vi "new FGGA TCP Packet_v3.1.vi"(0 "ID":string, 5 "Version":string, 7 "TCP Packet In":string, 9 "utc_time":u32, 12 "Data Array":string[](array[string])) -> (8 "TCP Binary Packet":string)   [LabVIEW 2014]
panel:
  out "array":string[](array[string])
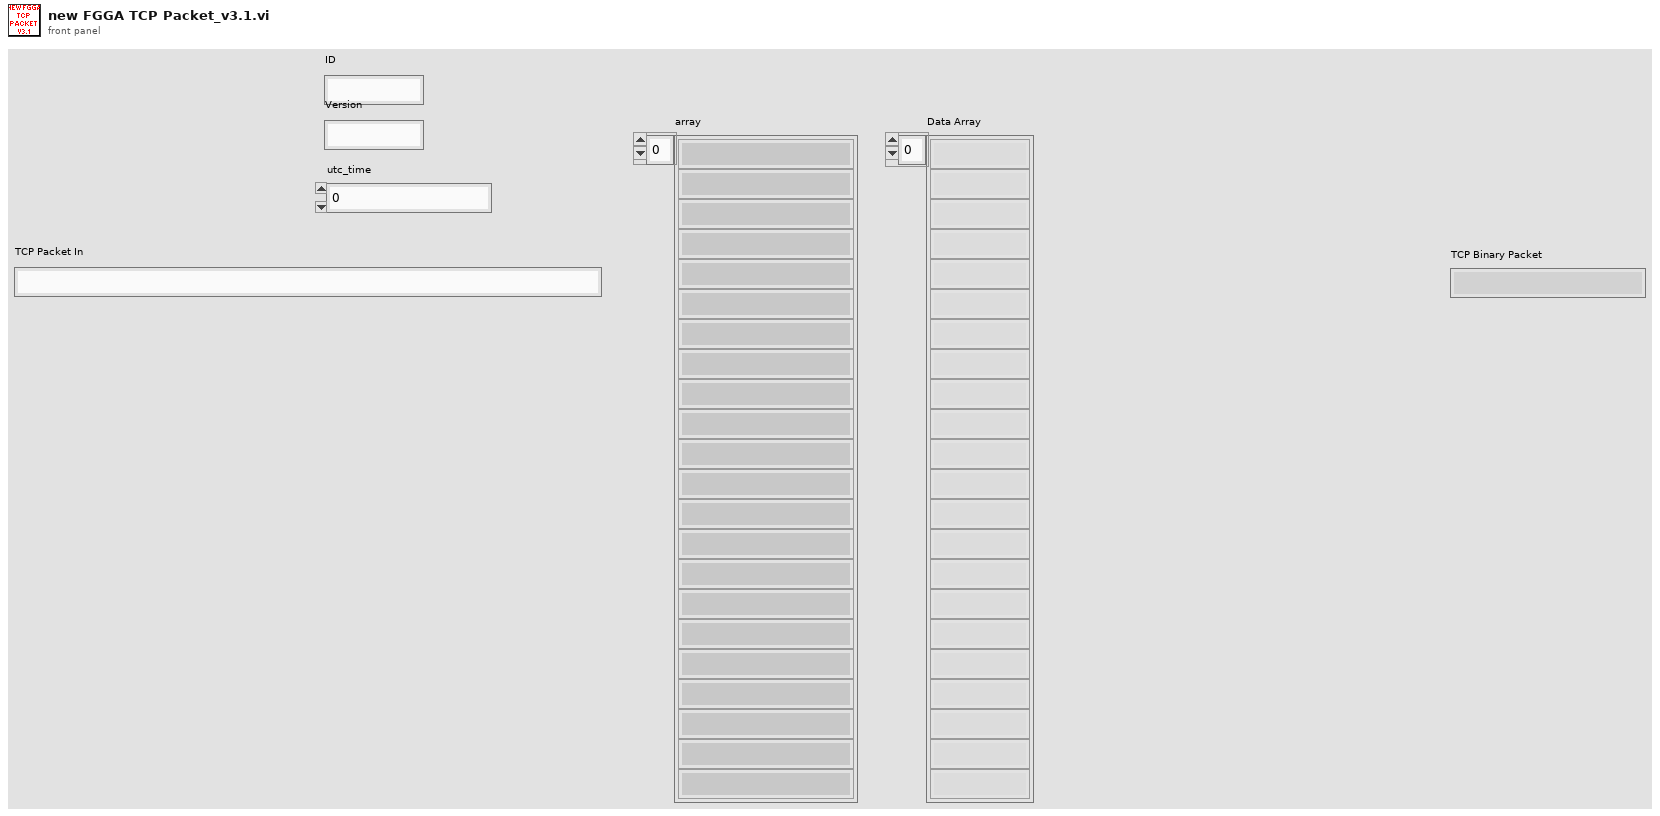
[diagram p1: front panel]
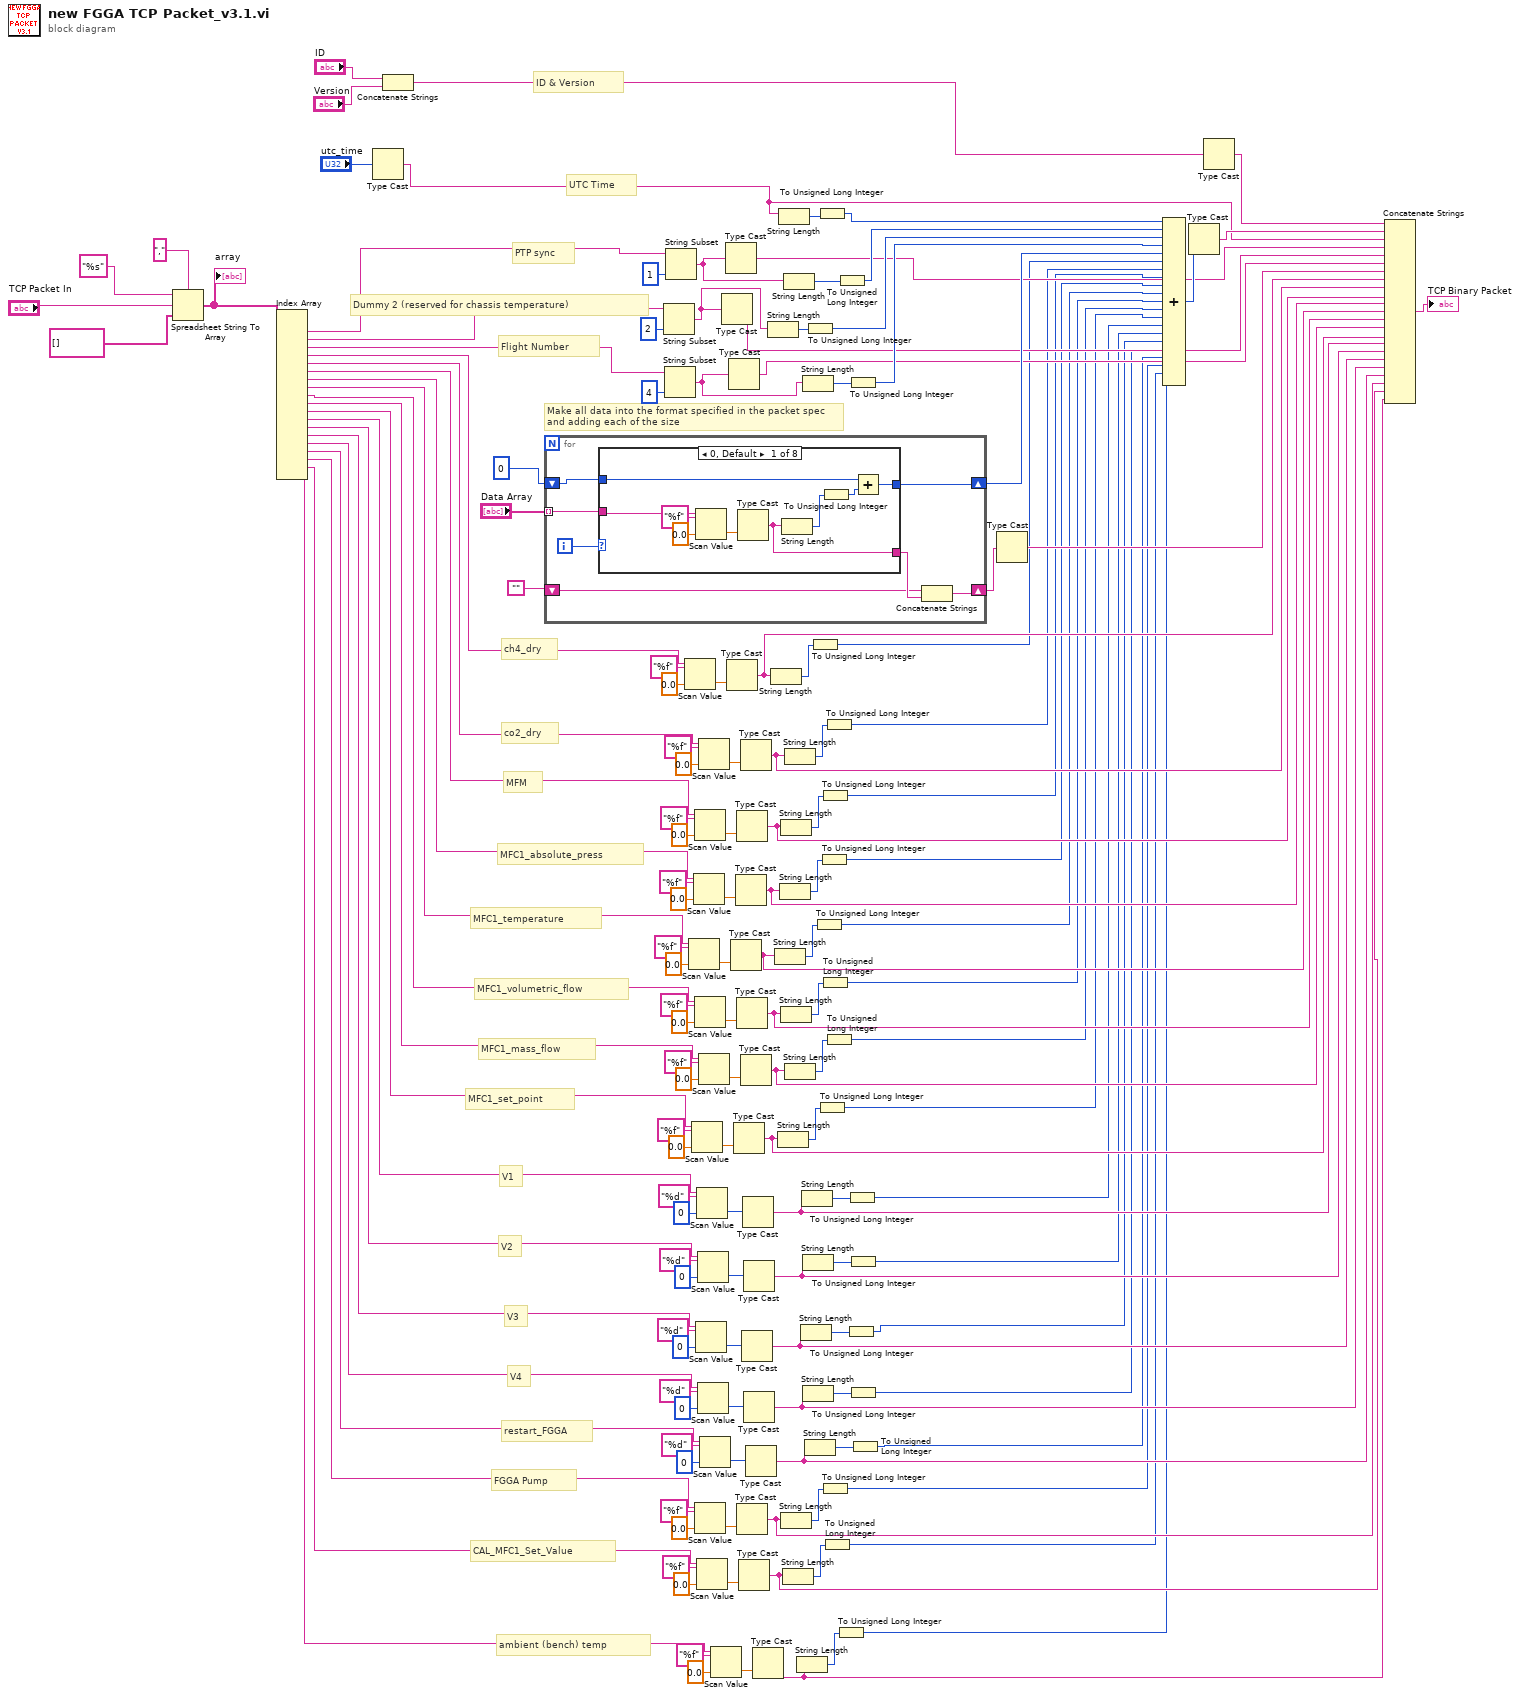
[diagram p0: block diagram]
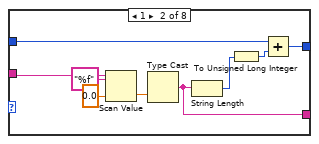
[diagram p2: hidden frame]
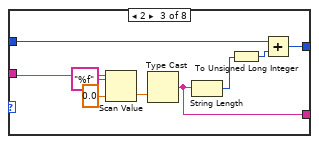
[diagram p3: hidden frame]
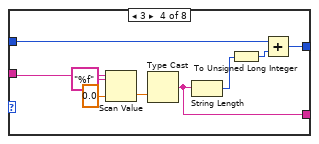
[diagram p4: hidden frame]
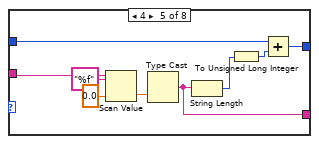
[diagram p5: hidden frame]
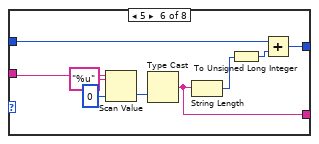
[diagram p6: hidden frame]
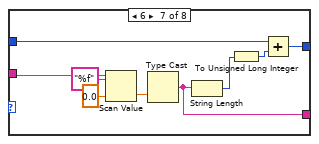
[diagram p7: hidden frame]
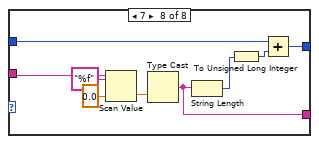
[diagram p8: hidden frame]
diagram:
  # "ambient (bench) temp"
  # "PTP sync"
  # "CAL_MFC1_Set_Value"
  # "FGGA Pump"
  # "restart_FGGA"
  # "V4"
  # "V3"
  # "V2"
  # "V1"
  # "MFC1_set_point"
  # "MFC1_mass_flow"
  # "MFC1_volumetric_flow"
  # "MFC1_temperature"
  # "MFC1_absolute_press"
  # "MFM"
  # "co2_dry"
  # "ch4_dry"
  # "Flight Number"
  # "Dummy 2 (reserved for chassis temperature)"
  # "UTC Time"
  # "ID & Version"
  # "Make all data into the format specified in the packet spec\nand adding each of the size"
  n1 = Spreadsheet String To Array(delimiter (Tab)=",", format string="%s", spreadsheet string="TCP Packet In", array type (2D Dbl)=string[] []) -> (array=w109:string[])
  "array" <- w109
  n2 = Index Array(array=w109) -> (element #1=w108:string, element #2=w107:string, element #3=w106:string, element #4=w105:string, element #5=w104:string, element #6=w79:string, element #7=w76:string, element #8=w73:string, element #9=w70:string, element #10=w67:string, element #11=w64:string, element #12=w57:string, element #13=w50:string, element #14=w27:string, element #15=w24:string, element #16=w21:string, element #17=w18:string, element #18=w15:string, element #19=w3:string)  [unwired: 19 in]
  n3 = Type Cast(x="utc_time") -> (*(type *) &x=w8:string)  [unwired: 1 in]
  n4 = Concatenate Strings("ID", "Version") -> (w10:string)
  n5 = for {
    tunnel: "Data Array" -> [w158] mode=indexing
    shift-right: [w156] -> w140
    shift-left: u32 0 -> [w157]
    shift-right: [w155] -> w129
    shift-left: "" -> [w153]
    i -> [w159]
    n6 = case shown="0, Default" w159 {
      tunnel: w158 -> [w166 w175 w184 w193 w202 w211 w220 w229]
      tunnel: w157 -> [w164 w173 w182 w191 w200 w209 w218 w227]
      tunnel: [w161 w170 w179 w188 w197 w206 w215 w224] -> w156
      tunnel: [w160 w169 w178 w187 w196 w205 w214 w223] -> w154
      frame 0, Default {
        n7 = Scan Value(string=w166, format string="%f", default (0 dbl)=sgl 0.0 ("default (0 I32)")) -> (value=w168:sgl)  [unwired: 1 out]
        n8 = Type Cast(x=w168) -> (*(type *) &x=w160:string)  [unwired: 1 in]
        n9 = String Length(string=w160) -> (length=w163:i32)
        n10 = To Unsigned Long Integer(number=w163) -> (unsigned 32bit integer=w162:u32)
        n11 = Add(x=w164, y=w162) -> (x+y=w161:u32)
      }
      frame 1 {
        n12 = Scan Value(string=w175, format string="%f", default (0 dbl)=sgl 0.0 ("default (0 I32)")) -> (value=w177:sgl)  [unwired: 1 out]
        n13 = Type Cast(x=w177) -> (*(type *) &x=w169:string)  [unwired: 1 in]
        n14 = String Length(string=w169) -> (length=w172:i32)
        n15 = To Unsigned Long Integer(number=w172) -> (unsigned 32bit integer=w171:u32)
        n16 = Add(x=w173, y=w171) -> (x+y=w170:u32)
      }
      frame 2 {
        n17 = Scan Value(string=w184, format string="%f", default (0 dbl)=sgl 0.0 ("default (0 I32)")) -> (value=w186:sgl)  [unwired: 1 out]
        n18 = Type Cast(x=w186) -> (*(type *) &x=w178:string)  [unwired: 1 in]
        n19 = String Length(string=w178) -> (length=w181:i32)
        n20 = To Unsigned Long Integer(number=w181) -> (unsigned 32bit integer=w180:u32)
        n21 = Add(x=w182, y=w180) -> (x+y=w179:u32)
      }
      frame 3 {
        n22 = Scan Value(string=w193, format string="%f", default (0 dbl)=sgl 0.0 ("default (0 I32)")) -> (value=w195:sgl)  [unwired: 1 out]
        n23 = Type Cast(x=w195) -> (*(type *) &x=w187:string)  [unwired: 1 in]
        n24 = String Length(string=w187) -> (length=w190:i32)
        n25 = To Unsigned Long Integer(number=w190) -> (unsigned 32bit integer=w189:u32)
        n26 = Add(x=w191, y=w189) -> (x+y=w188:u32)
      }
      frame 4 {
        n27 = Scan Value(string=w202, format string="%f", default (0 dbl)=sgl 0.0 ("default (0 I32)")) -> (value=w204:sgl)  [unwired: 1 out]
        n28 = Type Cast(x=w204) -> (*(type *) &x=w196:string)  [unwired: 1 in]
        n29 = String Length(string=w196) -> (length=w199:i32)
        n30 = To Unsigned Long Integer(number=w199) -> (unsigned 32bit integer=w198:u32)
        n31 = Add(x=w200, y=w198) -> (x+y=w197:u32)
      }
      frame 5 {
        n32 = Scan Value(string=w211, format string="%u", default (0 dbl)=u16 0 ("default (0 I32)")) -> (value=w213:u16)  [unwired: 1 out]
        n33 = Type Cast(x=w213) -> (*(type *) &x=w205:string)  [unwired: 1 in]
        n34 = String Length(string=w205) -> (length=w208:i32)
        n35 = To Unsigned Long Integer(number=w208) -> (unsigned 32bit integer=w207:u32)
        n36 = Add(x=w209, y=w207) -> (x+y=w206:u32)
      }
      frame 6 {
        n37 = Scan Value(string=w220, format string="%f", default (0 dbl)=sgl 0.0 ("default (0 I32)")) -> (value=w222:sgl)  [unwired: 1 out]
        n38 = Type Cast(x=w222) -> (*(type *) &x=w214:string)  [unwired: 1 in]
        n39 = String Length(string=w214) -> (length=w217:i32)
        n40 = To Unsigned Long Integer(number=w217) -> (unsigned 32bit integer=w216:u32)
        n41 = Add(x=w218, y=w216) -> (x+y=w215:u32)
      }
      frame 7 {
        n42 = Scan Value(string=w229, format string="%f", default (0 dbl)=sgl 0.0 ("default (0 I32)")) -> (value=w231:sgl)  [unwired: 1 out]
        n43 = Type Cast(x=w231) -> (*(type *) &x=w223:string)  [unwired: 1 in]
        n44 = String Length(string=w223) -> (length=w226:i32)
        n45 = To Unsigned Long Integer(number=w226) -> (unsigned 32bit integer=w225:u32)
        n46 = Add(x=w227, y=w225) -> (x+y=w224:u32)
      }
    }
    n47 = Concatenate Strings(w153, w154) -> (w155:string)
  }
  n48 = String Subset(string=w107, length (rest)=2 ("length (rest)")) -> (substring=w127:string)  [unwired: 1 in]
  n49 = String Subset(string=w106, length (rest)=4 ("length (rest)")) -> (substring=w133:string)  [unwired: 1 in]
  n50 = String Subset(string=w108, length (rest)=1 ("length (rest)")) -> (substring=w136:string)  [unwired: 1 in]
  n51 = Scan Value(string=w105, format string="%f", default (0 dbl)=sgl 0.0 ("default (0 I32)")) -> (value=w125:sgl)  [unwired: 1 out]
  n52 = Scan Value(string=w73, format string="%f", default (0 dbl)=sgl 0.0 ("default (0 I32)")) -> (value=w95:sgl)  [unwired: 1 out]
  n53 = Scan Value(string=w64, format string="%f", default (0 dbl)=sgl 0.0 ("default (0 I32)")) -> (value=w83:sgl)  [unwired: 1 out]
  n54 = Scan Value(string=w76, format string="%f", default (0 dbl)=sgl 0.0 ("default (0 I32)")) -> (value=w99:sgl)  [unwired: 1 out]
  n55 = Scan Value(string=w79, format string="%f", default (0 dbl)=sgl 0.0 ("default (0 I32)")) -> (value=w103:sgl)  [unwired: 1 out]
  n56 = Scan Value(string=w70, format string="%f", default (0 dbl)=sgl 0.0 ("default (0 I32)")) -> (value=w91:sgl)  [unwired: 1 out]
  n57 = Scan Value(string=w18, format string="%f", default (0 dbl)=sgl 0.0 ("default (0 I32)")) -> (value=w35:sgl)  [unwired: 1 out]
  n58 = Scan Value(string=w27, format string="%d", default (0 dbl)=u16 0 ("default (0 I32)")) -> (value=w44:u16)  [unwired: 1 out]
  n59 = Scan Value(string=w57, format string="%d", default (0 dbl)=u16 0 ("default (0 I32)")) -> (value=w58:u16)  [unwired: 1 out]
  n60 = Scan Value(string=w15, format string="%f", default (0 dbl)=sgl 0.0 ("default (0 I32)")) -> (value=w31:sgl)  [unwired: 1 out]
  n61 = Scan Value(string=w50, format string="%d", default (0 dbl)=u16 0 ("default (0 I32)")) -> (value=w51:u16)  [unwired: 1 out]
  n62 = Scan Value(string=w24, format string="%d", default (0 dbl)=u16 0 ("default (0 I32)")) -> (value=w40:u16)  [unwired: 1 out]
  n63 = Scan Value(string=w104, format string="%f", default (0 dbl)=sgl 0.0 ("default (0 I32)")) -> (value=w119:sgl)  [unwired: 1 out]
  n64 = Scan Value(string=w67, format string="%f", default (0 dbl)=sgl 0.0 ("default (0 I32)")) -> (value=w87:sgl)  [unwired: 1 out]
  n65 = Scan Value(string=w21, format string="%d", default (0 dbl)=u16 0 ("default (0 I32)")) -> (value=w36:u16)  [unwired: 1 out]
  n66 = Scan Value(string=w3, format string="%f", default (0 dbl)=sgl 0.0 ("default (0 I32)")) -> (value=w7:sgl)  [unwired: 1 out]
  n67 = Type Cast(x=w127) -> (*(type *) &x=w126:string)  [unwired: 1 in]
  n68 = Type Cast(x=w136) -> (*(type *) &x=w135:string)  [unwired: 1 in]
  n69 = Type Cast(x=w125) -> (*(type *) &x=w121:string)  [unwired: 1 in]
  n70 = Type Cast(x=w133) -> (*(type *) &x=w134:string)  [unwired: 1 in]
  n71 = Type Cast(x=w95) -> (*(type *) &x=w71:string)  [unwired: 1 in]
  n72 = Type Cast(x=w83) -> (*(type *) &x=w62:string)  [unwired: 1 in]
  n73 = Type Cast(x=w99) -> (*(type *) &x=w74:string)  [unwired: 1 in]
  n74 = Type Cast(x=w103) -> (*(type *) &x=w77:string)  [unwired: 1 in]
  n75 = Type Cast(x=w91) -> (*(type *) &x=w68:string)  [unwired: 1 in]
  n76 = Type Cast(x=w35) -> (*(type *) &x=w16:string)  [unwired: 1 in]
  n77 = Type Cast(x=w31) -> (*(type *) &x=w13:string)  [unwired: 1 in]
  n78 = Type Cast(x=w119) -> (*(type *) &x=w114:string)  [unwired: 1 in]
  n79 = Type Cast(x=w87) -> (*(type *) &x=w65:string)  [unwired: 1 in]
  n80 = Type Cast(x=w44) -> (*(type *) &x=w25:string)  [unwired: 1 in]
  n81 = Type Cast(x=w58) -> (*(type *) &x=w55:string)  [unwired: 1 in]
  n82 = Type Cast(x=w51) -> (*(type *) &x=w48:string)  [unwired: 1 in]
  n83 = Type Cast(x=w40) -> (*(type *) &x=w22:string)  [unwired: 1 in]
  n84 = Type Cast(x=w36) -> (*(type *) &x=w19:string)  [unwired: 1 in]
  n85 = Type Cast(x=w7) -> (*(type *) &x=w1:string)  [unwired: 1 in]
  n86 = String Length(string=w127) -> (length=w147:i32)
  n87 = String Length(string=w121) -> (length=w122:i32)
  n88 = String Length(string=w71) -> (length=w92:i32)
  n89 = String Length(string=w62) -> (length=w80:i32)
  n90 = String Length(string=w8) -> (length=w152:i32)
  n91 = String Length(string=w74) -> (length=w96:i32)
  n92 = String Length(string=w77) -> (length=w100:i32)
  n93 = String Length(string=w68) -> (length=w88:i32)
  n94 = String Length(string=w16) -> (length=w32:i32)
  n95 = String Length(string=w13) -> (length=w28:i32)
  n96 = String Length(string=w136) -> (length=w149:i32)
  n97 = String Length(string=w114) -> (length=w116:i32)
  n98 = String Length(string=w65) -> (length=w84:i32)
  n99 = String Length(string=w1) -> (length=w4:i32)
  n100 = String Length(string=w25) -> (length=w47:i32)
  n101 = String Length(string=w55) -> (length=w61:i32)
  n102 = String Length(string=w133) -> (length=w144:i32)
  n103 = String Length(string=w48) -> (length=w54:i32)
  n104 = String Length(string=w22) -> (length=w43:i32)
  n105 = To Unsigned Long Integer(number=w147) -> (unsigned 32bit integer=w146:u32)
  n106 = String Length(string=w19) -> (length=w39:i32)
  n107 = To Unsigned Long Integer(number=w122) -> (unsigned 32bit integer=w120:u32)
  n108 = To Unsigned Long Integer(number=w92) -> (unsigned 32bit integer=w72:u32)
  n109 = To Unsigned Long Integer(number=w152) -> (unsigned 32bit integer=w151:u32)
  n110 = To Unsigned Long Integer(number=w80) -> (unsigned 32bit integer=w63:u32)
  n111 = To Unsigned Long Integer(number=w96) -> (unsigned 32bit integer=w75:u32)
  n112 = To Unsigned Long Integer(number=w100) -> (unsigned 32bit integer=w78:u32)
  n113 = To Unsigned Long Integer(number=w88) -> (unsigned 32bit integer=w69:u32)
  n114 = To Unsigned Long Integer(number=w32) -> (unsigned 32bit integer=w17:u32)
  n115 = To Unsigned Long Integer(number=w28) -> (unsigned 32bit integer=w14:u32)
  n116 = To Unsigned Long Integer(number=w116) -> (unsigned 32bit integer=w115:u32)
  n117 = To Unsigned Long Integer(number=w84) -> (unsigned 32bit integer=w66:u32)
  n118 = To Unsigned Long Integer(number=w4) -> (unsigned 32bit integer=w2:u32)
  n119 = To Unsigned Long Integer(number=w149) -> (unsigned 32bit integer=w148:u32)
  n120 = To Unsigned Long Integer(number=w47) -> (unsigned 32bit integer=w26:u32)
  n121 = To Unsigned Long Integer(number=w61) -> (unsigned 32bit integer=w56:u32)
  n122 = To Unsigned Long Integer(number=w144) -> (unsigned 32bit integer=w143:u32)
  n123 = To Unsigned Long Integer(number=w54) -> (unsigned 32bit integer=w49:u32)
  n124 = To Unsigned Long Integer(number=w43) -> (unsigned 32bit integer=w23:u32)
  n125 = To Unsigned Long Integer(number=w39) -> (unsigned 32bit integer=w20:u32)
  n126 = Type Cast(x=w129) -> (*(type *) &x=w132:string)  [unwired: 1 in]
  n127 = Compound Arithmetic op=ADD(w151, w148, w146, w143, w140, w120, w115, w78, w75, w72, w69, w66, w63, w56, w49, w26, w23, w20, w17, w14, w2) -> (w138:u32)
  n128 = Type Cast(x=w138) -> (*(type *) &x=w137:string)  [unwired: 1 in]
  n129 = Type Cast(x=w10) -> (*(type *) &x=w139:string)  [unwired: 1 in]
  n130 = Concatenate Strings(w139, w137, w8, w135, w126, w134, w132, w121, w114, w77, w74, w71, w68, w65, w62, w55, w48, w25, w22, w19, w16, w13, w1) -> (→"TCP Binary Packet":string)
